vi "merFISH_email_title.vi"(2 "Probe number":i32, 3 "Item Names":string[][](array[string])) -> (0 "Title":string)   [LabVIEW 2015]
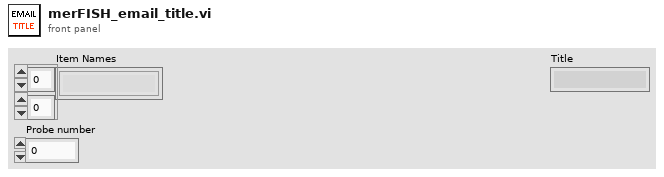
[diagram p1: front panel]
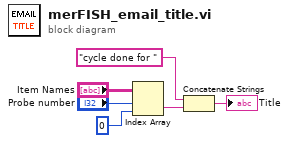
[diagram p0: block diagram]
diagram:
  n1 = Index Array(array="Item Names", index (row)="Probe number", index (col)=0 ("disabled index (col)")) -> (element=w3:string)
  n2 = Concatenate Strings("cycle done for " ("string"), w3) -> (→"Title":string)
